vi "K2420 current from multi-bias pulse.vi"() -> ()   [LabVIEW 2014]
uses:
  <vilib>/Utility/file.llb/Write To Spreadsheet File (string).vi
  Environmental Chamber LabVIEW and Instruments/Drivers and Software/LabVIEW 8.2 Drivers/keithley_24xx/Keithley 24XX/Public/Data/Read (Single Point).vi
  Environmental Chamber LabVIEW and Instruments/Drivers and Software/keithley_24xx/Keithley 24XX/Keithley 24XX.lvlib
panel:
  out "Save file path":path
  in  "Pulse amplitude (V)":dbl[](array[numeric])
  in  "Pulse time (min)":dbl=1.0 min=0.01 max=100.0
  out "Resistance (Ohm)":sgl
  out "Current (A)":sgl
  out "Voltage (V)":sgl
  out "XY Graph":cluster{"X":dbl[], "Y":dbl[]}[](graph)
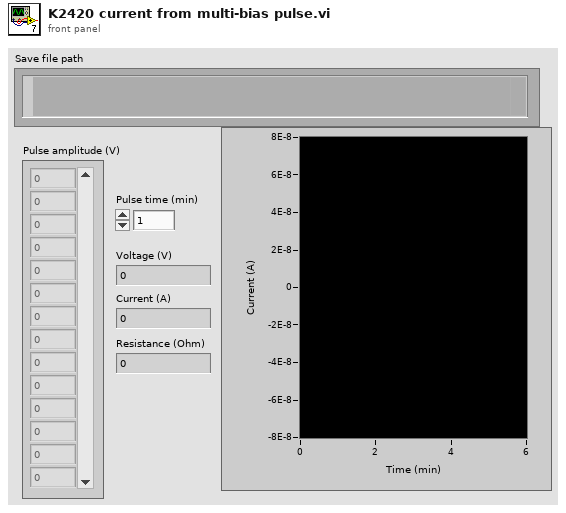
[diagram p1: front panel]
types:
  T1 = enum16{"open", "open or create", "create or replace", "create", "open (read only)"}
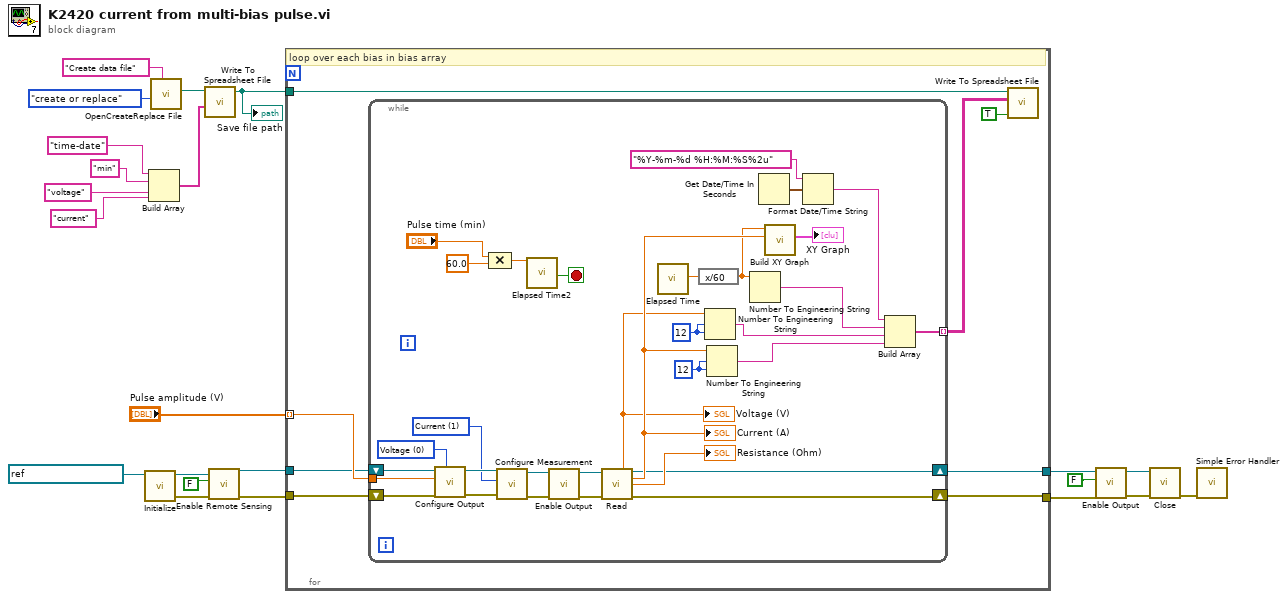
[diagram p0: block diagram]
diagram:
  n1 = call "Initialize.vi"("VISA resource name"=refnum<visa-resource-name> "GPIB1::24::INSTR") -> ("error out"=w18:errorcluster, "VISA resource name out"=w19:refnum<visa-resource-name>)  [unwired: 9 in]
  n2 = Build Array("time-date" ("note 2"), "min" ("note 2"), "voltage" ("note 2"), "current" ("note 2")) -> (w8:string[])
  n3 = call "OpenCreateReplace File.vi"("prompt"="Create data file", "function (open:0)"=T1."create or replace") -> ("new file path"=w9:path)  [unwired: 6 in, 3 out]
  n4 = call-poly <vilib>:"Write To Spreadsheet File.vi"("1D data"=w8, "file path (dialog if empty)"=w9) -> ("new file path (Not A Path if cancelled)"=w1:path)  [unwired: 6 in]
  "Save file path" <- w1
  n5 = call "Enable Remote Sensing.vi"("error in (no error)"=w18, "Enable Remote Sensing (T: Enable)"=FALSE ("4-wire?"), "VISA resource name"=w19) -> ("error out"=w4:errorcluster, "VISA resource name out"=w5:refnum<visa-resource-name>)  [unwired: 7 in]
  n6 = for {
    tunnel: "Pulse amplitude (V)" -> [w28] mode=indexing
    tunnel: w5 -> [w27]
    tunnel: w4 -> [w26]
    tunnel: [w30] -> w3
    tunnel: [w29] -> w2
    tunnel: w1 -> [w23]
    # "loop over each bias in bias array"
    n7 = while {
      tunnel: [w42] -> w24 mode=indexing
      tunnel: w28 -> [w39]
      shift-right: [w41] -> w30
      shift-left: w27 -> [w38]
      shift-right: [w40] -> w29
      shift-left: w26 -> [w37]
      stop <- w34 stop-if-true
      w58 = i16 12 ("width (-)")
      w49 = u16 0 items=["Voltage", "Current"] ("Source")
      w53 = u16 1 items=["Volts", "Current", "Resistance"] ("Measure")
      w47 = i16 12 ("width (-)")
      n8 = call "Configure Output.vi"("Source Mode  (0: Voltage)"=w49, "error in (no error)"=w37, "Output Level (0)"=w39, "VISA resource name"=w38) -> ("error out"=w55:errorcluster, "VISA resource name out"=w54:refnum<visa-resource-name>)  [unwired: 6 in]
      n9 = Compound Arithmetic op=MULTIPLY("Pulse time (min)", 60.0 ("value")) -> (w31:dbl)
      n10 = call "Configure Measurement.vi"("error in (no error)"=w55, "Function (0: Volts)"=w53, "VISA resource name"=w54) -> ("error out"=w56:errorcluster, "VISA resource name out"=w57:refnum<visa-resource-name>)  [unwired: 7 in]
      n11 = call "Elapsed Time2"("Time Target (s)"=w31) -> ("Time has Elapsed"=w34:bool)  [unwired: 11 in, 7 out]
      n12 = call "Enable Output.vi"("error in (no error)"=w56, "VISA resource name"=w57) -> ("error out"=w51:errorcluster, "VISA resource name out"=w50:refnum<visa-resource-name>)  [unwired: 8 in]
      n13 = call-poly "Read.vi"("VISA resource name"=w50, "error in (no error)"=w51) -> ("Voltage"=w60:sgl, "VISA resource name out"=w41:refnum<visa-resource-name>, "Current"=w61:sgl, "Resistance"=→"Resistance (Ohm)":sgl, "error out"=w40:errorcluster)  [unwired: 7 in, 2 out]
      "Voltage (V)" <- w60
      "Current (A)" <- w61
      n14 = call "Elapsed Time"() -> ("Elapsed Time (s)"=w35:dbl)  [unwired: 12 in, 7 out]
      n15 = expression code="x/60"(w35) -> (w36:dbl)
      n16 = Number To Engineering String(2:w47, 3:w47, 4:w60) -> (0:w48:string)  [unwired: 1 in]
      n17 = Number To Engineering String(2:w58, 3:w58, 4:w61) -> (0:w59:string)  [unwired: 1 in]
      n18 = Number To Engineering String ("elapsed time (min)")(4:w36) -> (0:w46:string)  [unwired: 3 in]
      n19 = Get Date/Time In Seconds() -> (seconds since 1Jan1904=w43:timestamp)
      n20 = call "Build XY Graph"("Y Input"=w61, "X Input"=w36) -> ("XY Graph"=→"XY Graph":cluster{"X":dbl[], "Y":dbl[]}[])  [unwired: 8 in, 1 out]
      n21 = Format Date/Time String(time format string (%c)="%Y-%m-%d %H:%M:%S%2u", seconds (now)=w43) -> (date/time string=w45:string)  [unwired: 1 in]
      n22 = Build Array(w45, w46, w48, w59) -> (w42:string[])
    }
    n23 = call-poly <vilib>:"Write To Spreadsheet File.vi"("append to file? (new file:F)"=TRUE, "2D data"=w24, "file path (dialog if empty)"=w23) -> ()  [unwired: 5 in, 1 out]
  }
  n24 = call "Enable Output.vi"("error in (no error)"=w2, "Enable Output (T: Enable)"=FALSE, "VISA resource name"=w3) -> ("error out"=w14:errorcluster, "VISA resource name out"=w16:refnum<visa-resource-name>)  [unwired: 7 in]
  n25 = call "Close.vi"("error in (no error)"=w14, "VISA resource name"=w16) -> ("error out"=w13:errorcluster)  [unwired: 9 in]
  n26 = call <vilib>:"Simple Error Handler.vi"("error in (no error)"=w13) -> ()  [unwired: 4 in, 5 out]
